vi "WebBrowser.vi"(3 "URL":string) -> ()   [LabVIEW 2015]
panel:
  in  "?":refnum<k7>(container)
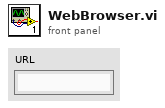
[diagram p1: front panel]
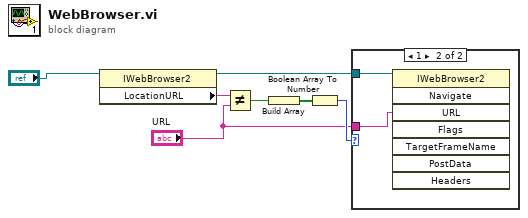
[diagram p0: block diagram]
diagram:
  n1 = property class="IWebBrowser2"(reference="?") -> (reference out=w7:refnum<k7>, "LocationURL"=w5:string)  [unwired: 1 in, 1 out]
  n2 = Not Equal?(x=w5, y="URL") -> (x != y?=w6:bool)
  n3 = Build Array(w6) -> (w4:bool[])
  n4 = Boolean Array To Number(Boolean array=w4) -> (number=w3:u32)
  n5 = case shown="1" w3 {
    tunnel: "URL" -> [_ w9]
    tunnel: w7 -> [_ w8]
    frame 0, Default {
    }
    frame 1 {
      n6 = invoke class="IWebBrowser2" method="Navigate"(reference=w8, "URL"=w9) -> ()  [unwired: 6 in, 8 out]
    }
  }
